vi "MoveXY.vi"() -> ()   [LabVIEW 2018]
panel:
  in  "Move":bool
  in  "stop":bool
  in  "X":dbl
  in  "Y":dbl
  in  "%Speed":dbl=10.0 format="%#_13g"
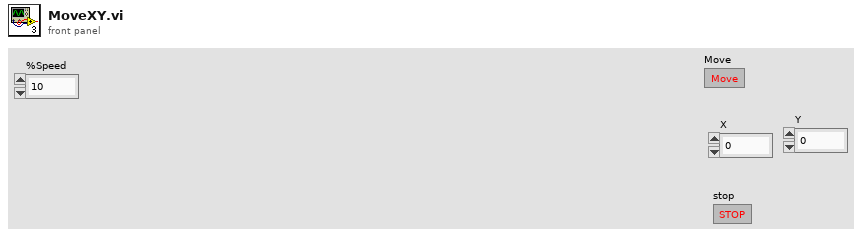
[diagram p1: front panel]
types:
  T1 = enum16{"Standard", "Buffered", "CRLF", "Immediate"}
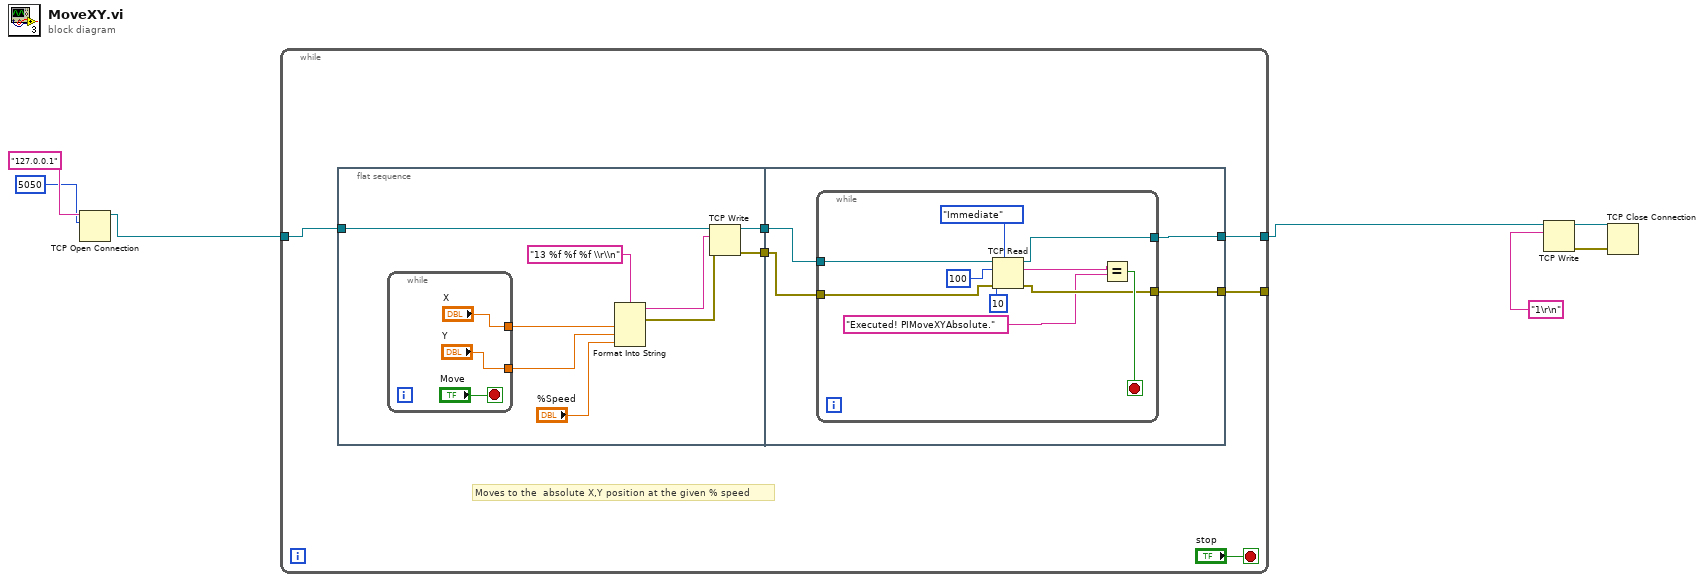
[diagram p0: block diagram]
diagram:
  n1 = TCP Open Connection(address="127.0.0.1", remote port or service name=u16 5050) -> (connection ID=w5:refnum<k5>)  [unwired: 3 in, 1 out]
  n2 = while {
    tunnel: [w10] -> _
    tunnel: w5 -> [w9]
    tunnel: [w11] -> w1
    stop <- "stop" stop-if-true
    # "Moves to the  absolute X,Y position at the given % speed"
    n3 = flat-sequence {
      tunnel: [w17] -> w13
      tunnel: [w16] -> w12
      tunnel: w9 -> [w15]
      tunnel: w13 -> [w28]
      tunnel: w12 -> [w29]
      tunnel: [w27] -> w11
      tunnel: [w26] -> w10
      frame #0 {
        n4 = while {
          tunnel: ["Y"] -> w21
          tunnel: ["X"] -> w14
          stop <- "Move" stop-if-true
        }
        n5 = Format Into String(format string="13 %f %f %f \\r\\n", w14, w21, "%Speed") -> (resulting string=w18:string, error out=w19:errorcluster)  [unwired: 2 in]
        n6 = TCP Write(connection ID=w15, data in=w18, error in (no error)=w19) -> (connection ID out=w17:refnum<k5>, error out=w16:errorcluster)  [unwired: 1 in, 1 out]
      }
      frame #1 {
        n7 = while {
          tunnel: w29 -> [w37]
          tunnel: [w33] -> w26
          tunnel: [w32] -> w27
          tunnel: w28 -> [w30]
          stop <- w34 stop-if-true
          n8 = TCP Read(connection ID=w30, bytes to read=100, error in (no error)=w37, 7:T1."Immediate" ("mode (standard)"), 9:10 ("timeout ms (25000)")) -> (connection ID out=w32:refnum<k5>, data out=w35:string, error out=w33:errorcluster)
          n9 = Equal?(x=w35, y="Executed! PIMoveXYAbsolute.") -> (x = y?=w34:bool)
        }
      }
    }
  }
  n10 = TCP Write(connection ID=w1, data in="1\r\n") -> (connection ID out=w3:refnum<k5>, error out=w4:errorcluster)  [unwired: 2 in, 1 out]
  n11 = TCP Close Connection(connection ID=w3, error in (no error)=w4) -> ()  [unwired: 1 in, 2 out]
